vi "Read analysis_date.vi"(8 "error in (no error)":errorcluster, 11 "Analysis in":refnum<class "Analysis.lvclass">) -> (0 "error out":errorcluster, 2 "analysis date":timestamp, 3 "Analysis out":refnum<class "Analysis.lvclass">)   [LabVIEW 2017, in "Analysis.lvclass"]
uses:
  Analysis.lvclass
  Analysis.lvclass/Analysis.ctl
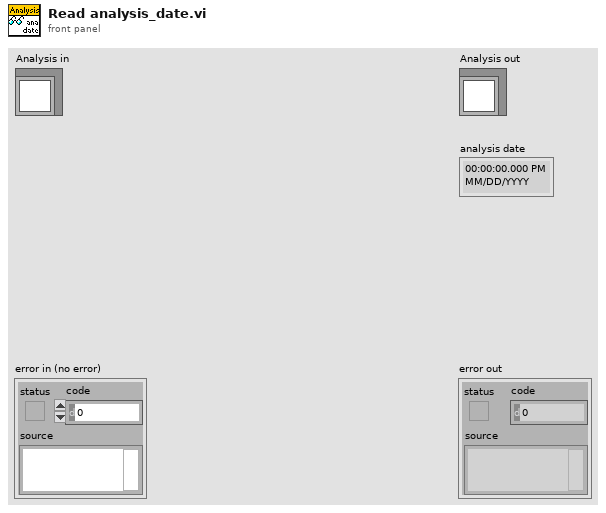
[diagram p1: front panel]
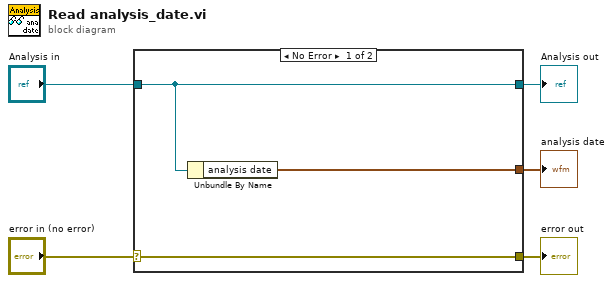
[diagram p0: block diagram]
diagram:
  n1 = case shown="No Error" "error in (no error)" {
    selector: "error in (no error)" -> [w8 w9]
    tunnel: [w8 w9] -> w4
    tunnel: [w7 w10] -> w2
    tunnel: "Analysis in" -> [w7 w10]
    tunnel: [w6 _] -> w1
    frame No Error {
      n2 = Unbundle By Name(w7) -> ("analysis date"=w6:timestamp)
    }
    frame Error {
    }
  }
  "error out" <- w4
  "Analysis out" <- w2
  "analysis date" <- w1
